vi "Create.vi"(8 "Error In":errorcluster) -> (0 "Error Out":errorcluster, 3 "Tag":refnum<class "Tag.lvclass">)   [LabVIEW 2017, in "Mustache.lvlib" / "Tokens.lvlib" / "Tag.lvclass"]
uses:
  Tag.lvclass
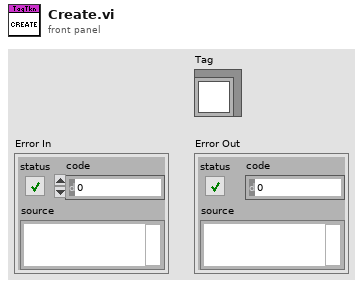
[diagram p1: front panel]
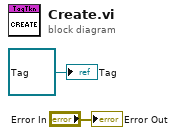
[diagram p0: block diagram]
diagram:
  "Tag" <- refnum<class "Tag.lvclass"> refnum ("Mustache.lvlib:Tokens.lvlib:Tag.lvclass")
  "Error Out" <- "Error In"
